vi "Get Statistics.vi"(8 "error in (no error)":errorcluster, 11 "Result Model in":refnum<class "Result Model.lvclass">) -> (0 "error out":errorcluster, 2 "Results":T1, 3 "Result Model out":refnum<class "Result Model.lvclass">)   [LabVIEW 2020, in "Result Model.lvclass"]
uses:
  Result Model.lvclass
  Statistics.ctl
  Result Model.lvclass/Result Model.ctl
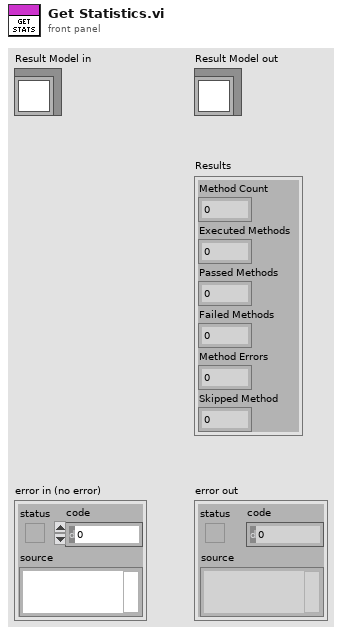
[diagram p1: front panel]
types:
  T1 = typedef "Result Model.lvclass/Statistics.ctl" = cluster{"Method Count":u32, "Executed Methods":u32, "Passed Methods":u32, "Failed Methods":u32, "Method Errors":u32, "Skipped Method":u32}
  T2 = typedef "Result.lvlib/Status.ctl" = enum16{"", "Passed", "Failed", "Error", "Skipped", "Setup Error", "Broken", "Teardown Error"}
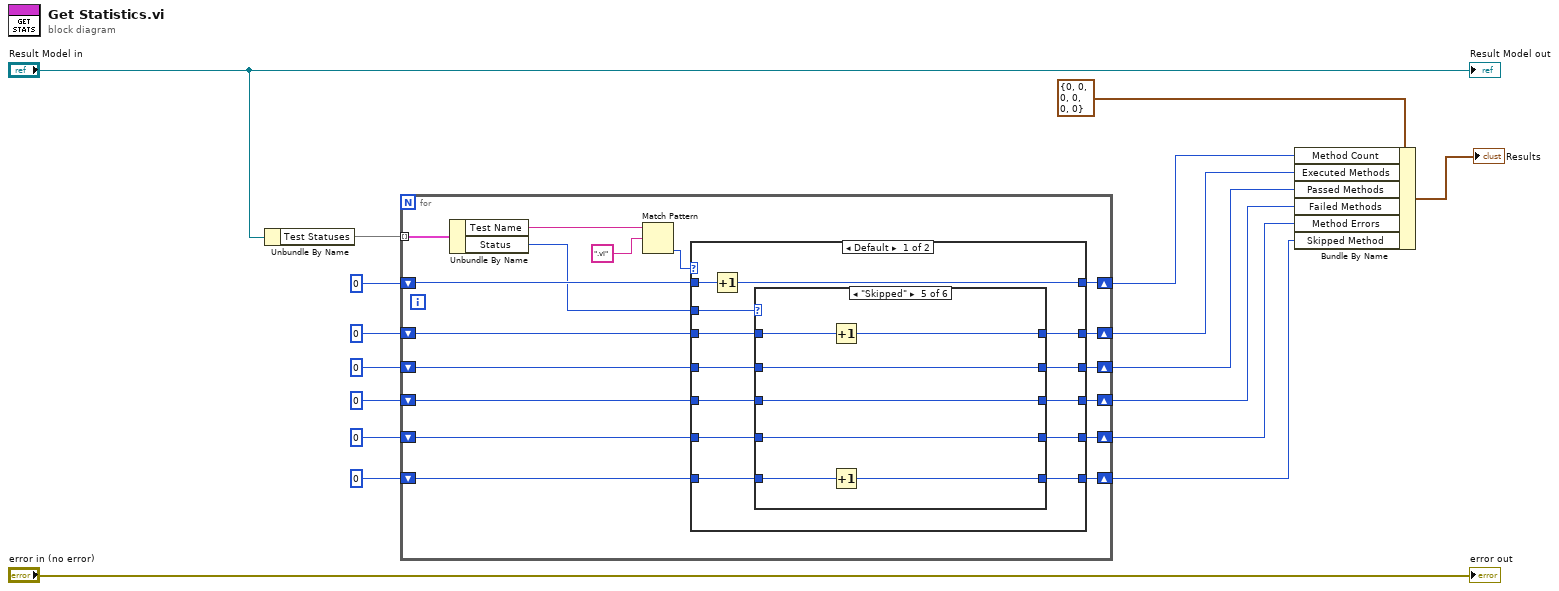
[diagram p0: block diagram]
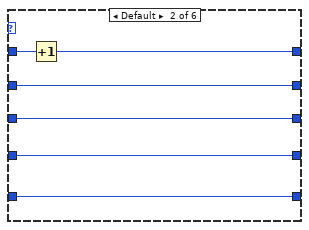
[diagram p3: hidden frame]
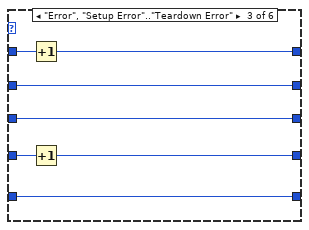
[diagram p4: hidden frame]
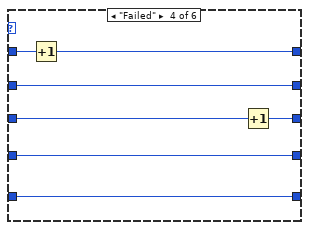
[diagram p5: hidden frame]
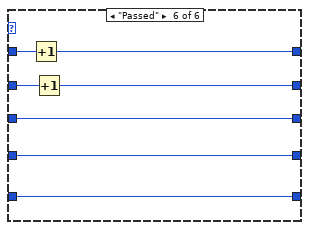
[diagram p6: hidden frame]
diagram:
  n1 = Unbundle By Name("Result Model in") -> ("Test Statuses"=w13:map{string, T2})
  n2 = for {
    tunnel: w13 -> [w34] mode=indexing
    shift-right: [w29] -> w11
    shift-left: u32 0 ("Method Count") -> [w30]
    shift-right: [w26] -> w9
    shift-left: u32 0 ("Method Count") -> [w27]
    shift-right: [w24] -> w7
    shift-left: u32 0 ("Method Count") -> [w25]
    shift-right: [w22] -> w5
    shift-left: u32 0 ("Method Count") -> [w23]
    shift-right: [w20] -> w3
    shift-left: u32 0 ("Method Count") -> [w21]
    shift-right: [w18] -> w1
    shift-left: u32 0 ("Method Count") -> [w19]
    n3 = Unbundle By Name(w34) -> ("Test Name"=w33:string, "Status"=w28:T2)
    n4 = Match Pattern(string=w33, regular expression=".vi") -> (offset past match=w31:i32)  [unwired: 1 in, 3 out]
    n5 = case shown="Default" w31 {
      tunnel: w30 -> [w47 w92]
      tunnel: [w46 w92] -> w29
      tunnel: w28 -> [w45 _]
      tunnel: w27 -> [w44 w91]
      tunnel: [w43 w91] -> w26
      tunnel: w25 -> [w42 w90]
      tunnel: [w41 w90] -> w24
      tunnel: w23 -> [w40 w89]
      tunnel: [w39 w89] -> w22
      tunnel: w21 -> [w38 w88]
      tunnel: [w37 w88] -> w20
      tunnel: w19 -> [w36 w87]
      tunnel: [w35 w87] -> w18
      frame Default {
        n6 = Increment(x=w47) -> (x+1=w46:u32)
        n7 = case shown="\"Skipped\"" w45 {
          tunnel: w44 -> [w52 w58 w65 w72 w79 w86]
          tunnel: [w52 w57 w64 w71 w78 w85] -> w43
          tunnel: w42 -> [w51 w56 w63 w70 w77 w84]
          tunnel: [w51 w56 w63 w70 w77 w83] -> w41
          tunnel: w40 -> [w50 w55 w62 w69 w76 w82]
          tunnel: [w50 w55 w62 w68 w76 w82] -> w39
          tunnel: w38 -> [w49 w54 w61 w67 w75 w81]
          tunnel: [w49 w54 w60 w67 w75 w81] -> w37
          tunnel: w36 -> [w48 w53 w59 w66 w74 w80]
          tunnel: [w48 w53 w59 w66 w73 w80] -> w35
          frame "" {
          }
          frame Default {
            n8 = Increment(x=w58) -> (x+1=w57:u32)
          }
          frame "Error", "Setup Error".."Teardown Error" {
            n9 = Increment(x=w65) -> (x+1=w64:u32)
            n10 = Increment(x=w61) -> (x+1=w60:u32)
          }
          frame "Failed" {
            n11 = Increment(x=w72) -> (x+1=w71:u32)
            n12 = Increment(x=w69) -> (x+1=w68:u32)
          }
          frame "Skipped" {
            n13 = Increment(x=w79) -> (x+1=w78:u32)
            n14 = Increment(x=w74) -> (x+1=w73:u32)
          }
          frame "Passed" {
            n15 = Increment(x=w86) -> (x+1=w85:u32)
            n16 = Increment(x=w84) -> (x+1=w83:u32)
          }
        }
      }
      frame -1 {
      }
    }
  }
  n17 = Bundle By Name(cluster=T1 {"Method Count"=0, "Executed Methods"=0, "Passed Methods"=0, "Failed Methods"=0, "Method Errors"=0, "Skipped Method"=0} ("Results"), "Method Count"=w11, "Executed Methods"=w9, "Passed Methods"=w7, "Failed Methods"=w5, "Method Errors"=w3, "Skipped Method"=w1) -> (→"Results":T1)
  "error out" <- "error in (no error)"
  "Result Model out" <- "Result Model in"
